vi "_RT_CtrlLoop_Pressure_GetResponseValue.vi"(8 "error in":errorcluster, 11 "Response Str":string) -> (0 "error out":errorcluster, 3 "Value":string)   [LabVIEW 2018]
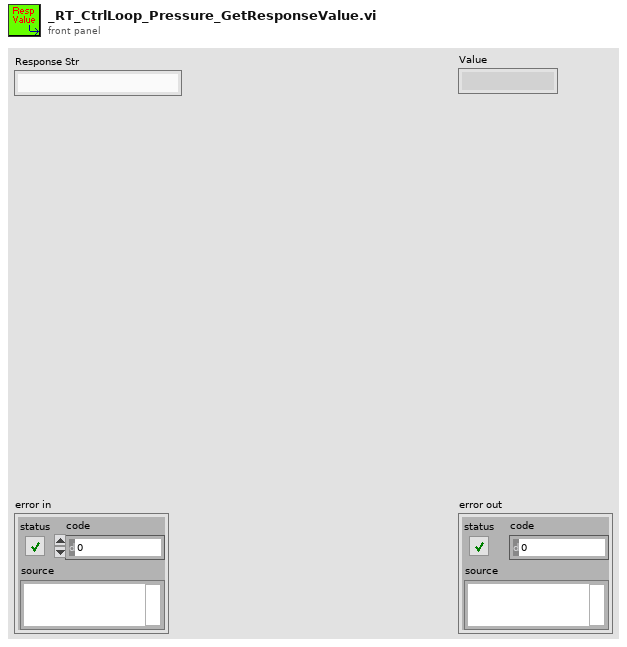
[diagram p1: front panel]
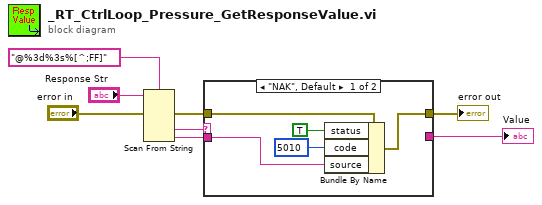
[diagram p0: block diagram]
diagram:
  n1 = Scan From String(format string="@%3d%3s%[^;FF]", input string="Response Str", error in="error in") -> (error out=w5:errorcluster, output 2=w1:string, output 3=w2:string)  [unwired: 5 in, 2 out]
  n2 = case shown="\"NAK\", Default" w1 {
    tunnel: w5 -> [w13 w15]
    tunnel: [w10 w15] -> w4
    tunnel: [_ w14] -> w3
    tunnel: w2 -> [w9 w14]
    frame "NAK", Default {
      n3 = Bundle By Name(cluster=w13, "status"=TRUE, "code"=5010, "source"=w9) -> (w10:errorcluster)
    }
    frame "ACK" {
    }
  }
  "error out" <- w4
  "Value" <- w3
